vi "Encoders.vi"(7 "error in (no error) 2":errorcluster, 8 "error in (no error)":errorcluster, 10 "Left Encoder":T1={"DevStatus"={"status"=FALSE, "code"=0, "source"=""}, "EncoderIndex"=enum."Invalid", "CounterIndex"=enum."Ctr 1", "DistancePerCount"=2.0, "Decoding Type"=enum."4x"}, 11 "Right Encoder":T1={"DevStatus"={"status"=FALSE, "code"=0, "source"=""}, "EncoderIndex"=enum."Invalid", "CounterIndex"=enum."Ctr 1", "DistancePerCount"=2.0, "Decoding Type"=enum."4x"}) -> ()   [LabVIEW 2011]
uses:
  <vilib>/Rock Robotics/WPI/Encoder/WPI_EncoderDevRef.ctl
  <vilib>/Rock Robotics/SystemInterfaces/Encoder/FPGA_EncoderIdx.ctl
  <vilib>/Rock Robotics/SystemInterfaces/Counter/FPGA_CounterCtrSystemIndex.ctl
  <vilib>/Rock Robotics/WPI/Encoder/WPI_EncoderType.ctl
  <vilib>/Rock Robotics/WPI/DriverStation/DriverStationLCD/WPI_DriverStationLCDLCDLine.ctl
  Robot Global Data.vi
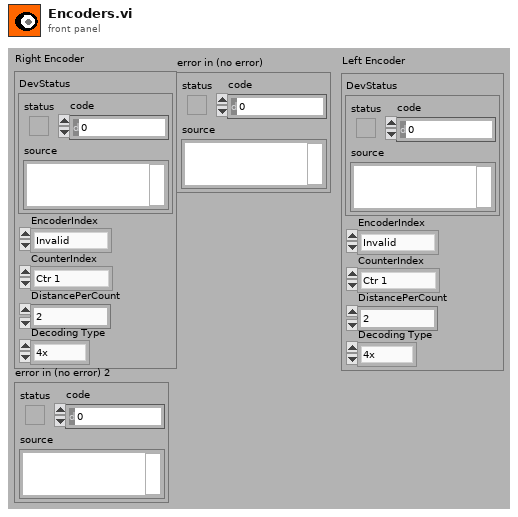
[diagram p1: front panel]
types:
  T1 = typedef "WPI_EncoderDevRef.ctl" = cluster{"DevStatus":errorcluster, "EncoderIndex":T2, "CounterIndex":T3, "DistancePerCount":dbl, "Decoding Type":T4}
  T2 = typedef "FPGA_EncoderIdx.ctl" = enum8{"Enc 0", "Enc 1", "Enc 2", "Enc 3", "Invalid"}
  T3 = typedef "FPGA_CounterCtrSystemIndex.ctl" = enum8{"Ctr 0", "Ctr 1", "Ctr 2", "Ctr 3", "Ctr 4", "Ctr 5", "Ctr 6", "Ctr 7", "Invalid"}
  T4 = typedef "WPI_EncoderType.ctl" = enum16{"1x", "2x", "4x"}
  T5 = typedef "WPI_DriverStationLCDLCDLine.ctl" = enum16{"Main - Line 1", "User - Line 2", "User - Line 3", "User - Line 4", "User - Line 5", "User - Line 6"}
  T6 = typedef "WPI_JoystickDevRef.ctl" = cluster{"Device":T7}
  T7 = typedef "WPI_JoystickDeviceEnum.ctl" = enum16{"USB 1", "USB 2", "USB 3", "USB 4", "Kinect 1", "Kinect 2"}
  T8 = cluster{"axis 1 (x)":dbl, "axis 2 (y)":dbl, "axis 3 (throttle)":dbl, "axis 4":dbl, "axis 5":dbl, "axis 6":dbl}
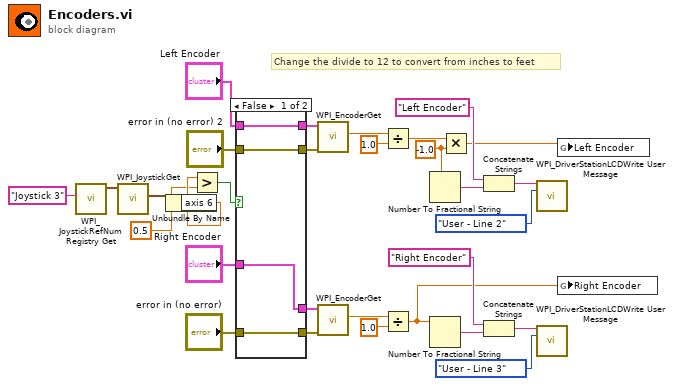
[diagram p0: block diagram]
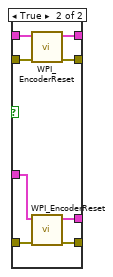
[diagram p2: hidden frame]
diagram:
  w3 = -1.0 ("y")
  # "Change the divide to 12 to convert from inches to feet"
  n1 = call <vilib>:"WPI_JoystickRefNum Registry Get.vi"("refnum name"="Joystick 3") -> ("JoystickDevRef"=w21:T6)  [unwired: 1 in, 9 out]
  n2 = call <vilib>:"WPI_JoystickGet.vi"("JoystickDevRef"=w21) -> ("Axes"=w7:T8)  [unwired: 1 in, 5 out]
  n3 = Unbundle By Name(w7) -> ("axis 6"=w6:dbl)
  n4 = Greater?(x=w6, y=0.5) -> (0:w4:bool)
  n5 = case shown="False" w4 {
    tunnel: "Right Encoder" -> [w34 w42]
    tunnel: "error in (no error)" -> [w33 w41]
    tunnel: [w34 w40] -> w28
    tunnel: [w33 w39] -> w27
    tunnel: [w31 w38] -> w23
    tunnel: [w32 w37] -> w24
    tunnel: "error in (no error) 2" -> [w31 w36]
    tunnel: "Left Encoder" -> [w32 w35]
    frame False {
    }
    frame True {
      n6 = call <vilib>:"WPI_EncoderReset.vi"("error in (no error)"=w36, "EncoderDevRef"=w35) -> ("error out"=w38:errorcluster, "EncoderDevRef"=w37:T1)  [unwired: 8 out]
      n7 = call <vilib>:"WPI_EncoderReset.vi"("error in (no error)"=w41, "EncoderDevRef"=w42) -> ("error out"=w39:errorcluster, "EncoderDevRef"=w40:T1)  [unwired: 8 out]
    }
  }
  n8 = call <vilib>:"WPI_EncoderGet.vi"("error in (no error)"=w23, "EncoderDevRef"=w24) -> ("Distance"=w19:dbl)  [unwired: 9 out]
  n9 = call <vilib>:"WPI_EncoderGet.vi"("error in (no error)"=w27, "EncoderDevRef"=w28) -> ("Distance"=w20:dbl)  [unwired: 9 out]
  n10 = Divide(x=w19, y=1.0) -> (x/y=w14:dbl)
  n11 = Divide(x=w20, y=1.0) -> (x/y=w1:dbl)
  n12 = Number To Fractional String(number=w3) -> (F-format string=w13:string)  [unwired: 3 out]
  n13 = Number To Fractional String(number=w1) -> (F-format string=w11:string)  [unwired: 3 out]
  n14 = Multiply(x=w14, y=w3) -> (x*y=w2:dbl)
  n15 = Concatenate Strings("Left Encoder" ("string"), w13) -> (w8:string)
  n16 = Concatenate Strings("Right Encoder" ("string"), w11) -> (w9:string)
  n17 = call <vilib>:"WPI_DriverStationLCDWrite User Message.vi"("line text"=w8, "line"=WPI_DriverStationLCDLCDLine."User - Line 2") -> ()  [unwired: 3 in, 11 out]
  n18 = call <vilib>:"WPI_DriverStationLCDWrite User Message.vi"("line text"=w9, "line"=WPI_DriverStationLCDLCDLine."User - Line 3") -> ()  [unwired: 3 in, 11 out]
  n19 = global write "Robot Global Data.vi" "Left Encoder"(w2) -> ()
  n20 = global write "Robot Global Data.vi" "Right Encoder"(w1) -> ()
